vi "Read Radius.vi"(8 "error in (no error)":errorcluster, 11 "Circle Collider in":refnum<class "Circle Collider.lvclass">) -> (0 "error out":errorcluster, 2 "Radius":i16, 3 "Circle Collider out":refnum<class "Circle Collider.lvclass">)   [LabVIEW 2022 SP3, in "Circle Collider.lvclass"]
uses:
  Circle Collider.lvclass
  Circle Collider.lvclass/Circle Collider.ctl
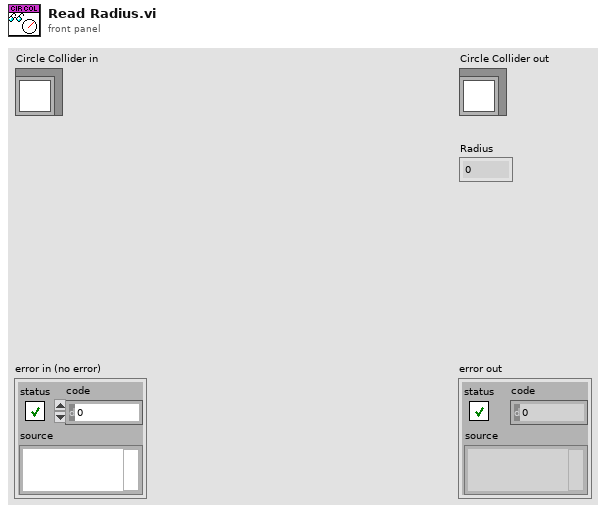
[diagram p1: front panel]
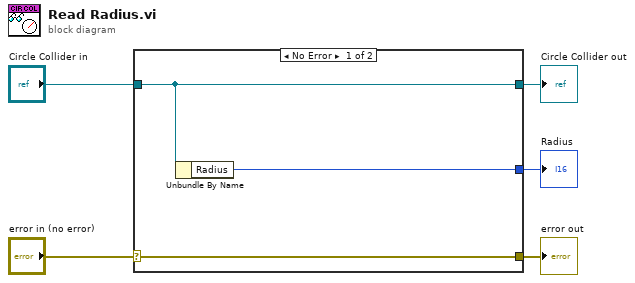
[diagram p0: block diagram]
diagram:
  n1 = case shown="No Error" "error in (no error)" {
    selector: "error in (no error)" -> [w8 w9]
    tunnel: [w8 w9] -> w4
    tunnel: [w7 w10] -> w2
    tunnel: "Circle Collider in" -> [w7 w10]
    tunnel: [w6 _] -> w1
    frame No Error {
      n2 = Unbundle By Name(w7) -> ("Radius"=w6:i16)
    }
    frame Error {
    }
  }
  "error out" <- w4
  "Circle Collider out" <- w2
  "Radius" <- w1
